vi "Pass If Equal 1D Array (String).vi"(6 "case sensitive? (T)":bool=TRUE, 8 "error in (no error)":errorcluster, 9 "actual":string[](array[string]), 10 "expected":string[](array[string]), 11 "TestCase in":refnum<class "TestCase.lvclass">) -> (0 "error out":errorcluster, 3 "TestCase out":refnum<class "TestCase.lvclass">)   [LabVIEW 2015, in "VITAC.lvlib"]
doc: "Compares two 1D string arrays and returns a pass if arrays are equal.\n\nThe results string will identify the strings that don't match as well as the array index.\n\nString comparison is optionally case-sensitive.\n\nDefault is case-sensitive match."
uses:
  VITAC.lvlib
  <vilib>/addons/_JKI Toolkits/VI Tester/TestCase.llb/TestCase.lvclass
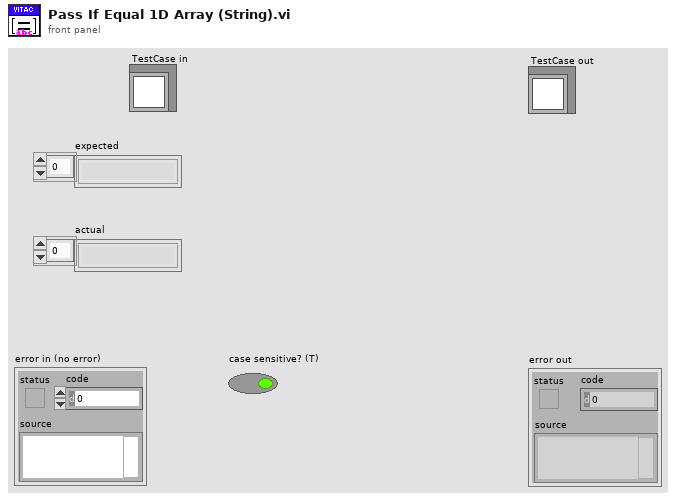
[diagram p1: front panel]
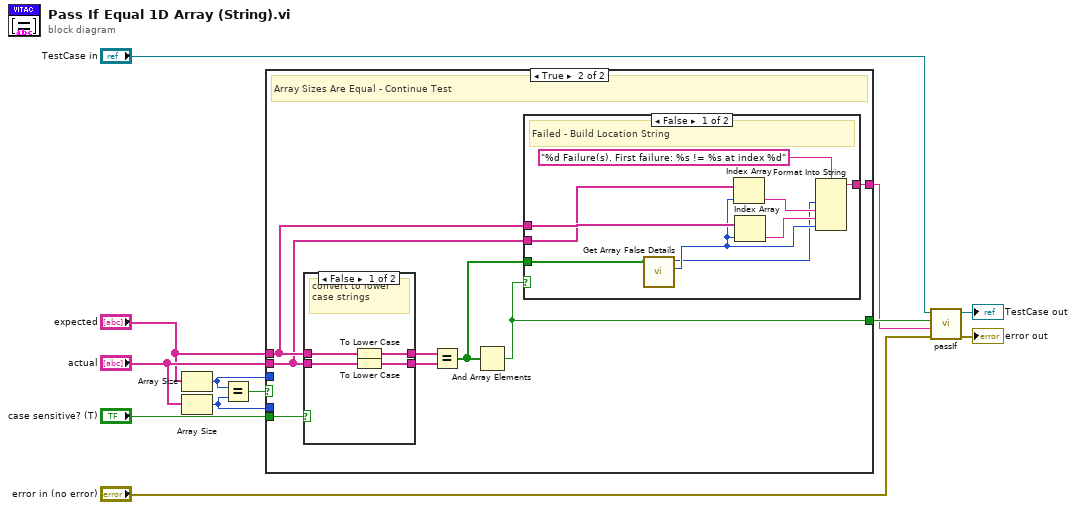
[diagram p0: block diagram]
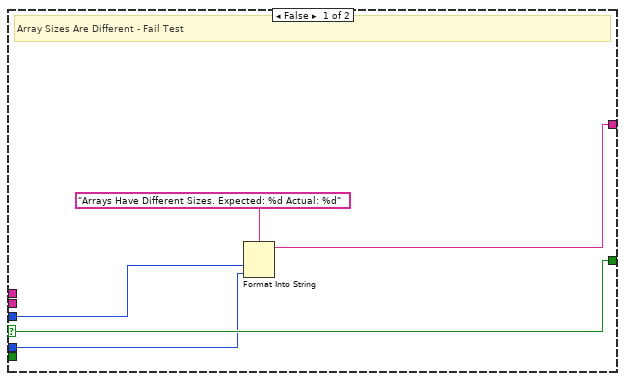
[diagram p2: hidden frame]
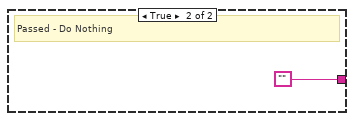
[diagram p4: hidden frame]
diagram:
  n1 = Array Size(array="expected") -> (size(s)=w5:i32)
  n2 = Array Size(array="actual") -> (size(s)=w4:i32)
  n3 = Equal?(x=w5, y=w4) -> (x = y?=w6:bool)
  n4 = case shown="True" w6 {
    selector: w6 -> [w17 _]
    tunnel: "case sensitive? (T)" -> [_ w22]
    tunnel: [w17 w23] -> w8
    tunnel: [w13 w25] -> w7
    tunnel: "expected" -> [_ w20]
    tunnel: "actual" -> [_ w19]
    tunnel: w5 -> [w14 _]
    tunnel: w4 -> [w15 _]
    frame False {
      # "Array Sizes Are Different - Fail Test"
      n5 = Format Into String(format string="Arrays Have Different Sizes. Expected: %d Actual: %d", w14, w15) -> (resulting string=w13:string)  [unwired: 2 in, 1 out]
    }
    frame True {
      # "Array Sizes Are Equal - Continue Test"
      n6 = case shown="False" w22 {
        tunnel: [w27 w31] -> w21
        tunnel: w20 -> [w29 w31]
        tunnel: w19 -> [w28 w30]
        tunnel: [w26 w30] -> w18
        frame False {
          # "convert to lower\ncase strings"
          n7 = To Lower Case(string=w29) -> (all lower case string=w27:string[])
          n8 = To Lower Case(string=w28) -> (all lower case string=w26:string[])
        }
        frame True {
        }
      }
      n9 = Equal?(x=w21, y=w18) -> (x = y?=w24:bool[])
      n10 = And Array Elements(Boolean array=w24) -> (logical AND=w23:bool)
      n11 = case shown="False" w23 {
        tunnel: w24 -> [w34 _]
        tunnel: w20 -> [w36 _]
        tunnel: w19 -> [w35 _]
        tunnel: [w37 ""] -> w25
        frame False {
          # "Failed - Build Location String"
          n12 = call "Get Array False Details.vi"("Array"=w34) -> ("First False"=w33:i32, "Count"=w32:i16)  [unwired: 9 in]
          n13 = Index Array(array=w35, index=w33) -> (element=w39:string)
          n14 = Index Array(array=w36, index=w33) -> (element=w38:string)
          n15 = Format Into String(format string="%d Failure(s). First failure: %s != %s at index %d", w32, w39, w38, w33) -> (resulting string=w37:string)  [unwired: 2 in, 1 out]
        }
        frame True {
          # "Passed - Do Nothing"
        }
      }
    }
  }
  n16 = call-dynamic "passIf.vi"("error in (no error)"="error in (no error)", "message (\"\")"=w7, "pass"=w8, "TestCase in"="TestCase in") -> ("error out"=→"error out":errorcluster, "TestCase out"=→"TestCase out":refnum<class "TestCase.lvclass">)  [unwired: 6 in]
